vi "File Directory Path.vi"(6 "Mode (All)":i32(ring) items=["All", "Without Attributes"], 8 "error in (no error)":errorcluster, 9 "Directory (\"D:\\user\\data\")":string="D:\\user\\data", 10 "Read (Subdirectories and Files)":i32(ring) items=["Subdirectories and Files", "Subdirectories"], 11 "VISA resource name":refnum<visa-resource-name>) -> (0 "error out":errorcluster, 2 "Output":string, 3 "VISA resource name out":refnum<visa-resource-name>)   [LabVIEW 2020, in "Rohde&Schwarz CMXP Base.lvlib"]
doc: "This VI reads out the contents of the current of a specified directory. If no directory is specified, the default directory selected with the MMEM:CDIR command.\n\nAttribute:\n-\n\nRemote-control commands:\nMMEMory:CATalog?\nMMEMory:DCATalog?"
uses:
  <instrlib>/Rohde&Schwarz CMXP Base/Rohde&Schwarz CMXP Base.lvlib
  <instrlib>/Rohde&Schwarz CMXP Base/Private/rsidr_core.llb/rsidr_core.lvlib
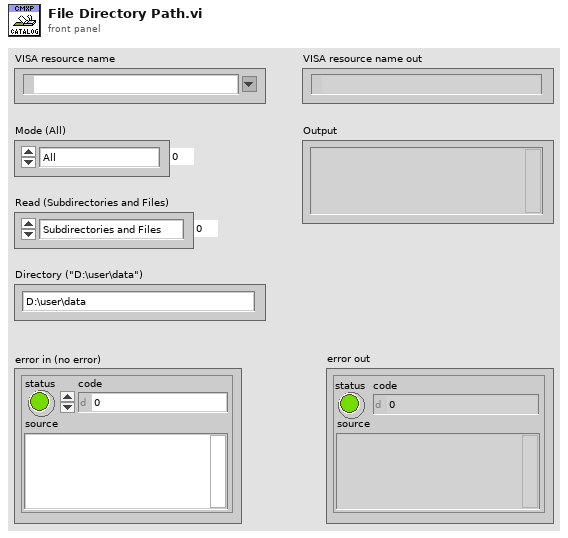
[diagram p1: front panel]
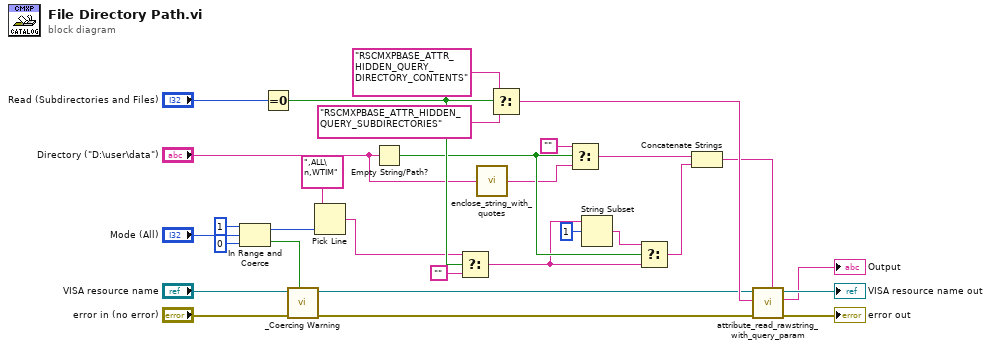
[diagram p0: block diagram]
diagram:
  n1 = In Range and Coerce(upper limit=1, x="Mode (All)", lower limit=0) -> (coerced(x)=w22:i32, In Range?=w17:bool)
  n2 = Equal To 0?(x="Read (Subdirectories and Files)") -> (x = 0?=w13:bool)
  n3 = call <instrlib>:"_Coercing Warning.vi"("In Range?"=w17, "error in (no error)"="error in (no error)", "VISA resource name"="VISA resource name") -> ("error out"=w19:errorcluster, "VISA resource name out"=w18:refnum<visa-resource-name>)  [unwired: 7 in]
  n4 = Pick Line(multi-line string=",ALL\n,WTIM", line index=w22) -> (output string=w9:string)  [unwired: 1 in]
  n5 = Empty String/Path?(string/path="Directory (\"D:\\user\\data\")") -> (empty?=w12:bool)
  n6 = Select(t=w9, s=w13, f="" ("Empty String Constant")) -> (s? t:f=w7:string)
  n7 = call <instrlib>:"enclose_string_with_quotes.vi"("String to enclose"="Directory (\"D:\\user\\data\")") -> ("String out"=w1:string)  [unwired: 4 in]
  n8 = Select(t="RSCMXPBASE_ATTR_HIDDEN_QUERY_DIRECTORY_CONTENTS", s=w13, f="RSCMXPBASE_ATTR_HIDDEN_QUERY_SUBDIRECTORIES") -> (s? t:f=w26:string)
  n9 = Select(t="" ("Empty String Constant"), s=w12, f=w1) -> (s? t:f=w25:string)
  n10 = String Subset(string=w7, offset (0)=1) -> (substring=w6:string)  [unwired: 1 in]
  n11 = Select(t=w6, s=w12, f=w7) -> (s? t:f=w10:string)
  n12 = Concatenate Strings(w25, w10) -> (w11:string)
  n13 = call <instrlib>:"attribute_read_rawstring_with_query_param.vi"("Query Parameter (None)"=w11, "error in"=w19, "Attribute ID"=w26, "VISA resource name"=w18) -> ("error out"=→"error out":errorcluster, "RawString out"=→"Output":string, "VISA resource name out"=→"VISA resource name out":refnum<visa-resource-name>)  [unwired: 5 in]
